vi "Configure Trigger.vi"(4 "impedence":enum16{"50 Ohm", "1 kOhm"}(ring), 6 "threshold (V)":dbl=1.0 min=0.9 max=1.6, 8 "error in (no error)":errorcluster, 9 "trigger source":T2, 10 "trigger mode":T1 items=["Single", "Continuous", "Gated", "Burst"], 11 "VISA resource name":refnum<visa-resource-name>) -> (0 "error out":errorcluster, 3 "VISA resource name out":refnum<visa-resource-name>)   [LabVIEW 2019, in "Pulse Rider PG-1000.lvlib"]
doc: "Configures the triggering settings of the instrument."
uses:
  <instrlib>/LV_PulseRiderPG1000/Pulse Rider PG-1000.lvlib
  <instrlib>/LV_PulseRiderPG1000/Public/Configure/Trigger/Trigger Source.ctl
  <instrlib>/LV_PulseRiderPG1000/Public/Configure/Trigger/Trigger Mode.ctl
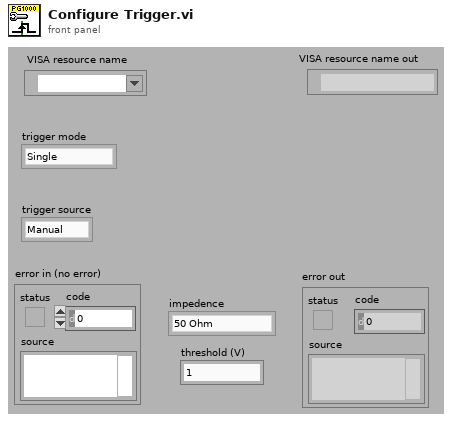
[diagram p1: front panel]
types:
  T1 = typedef "Pulse Rider PG-1000.lvlib/Trigger Mode.ctl" = u16
  T2 = typedef "Pulse Rider PG-1000.lvlib/Trigger Source.ctl" = enum16{"Manual", "External", "Timer"}
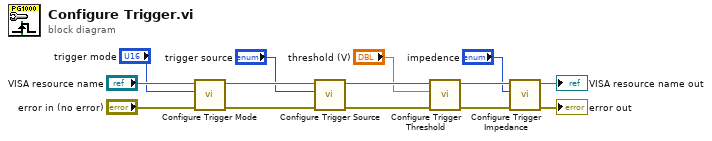
[diagram p0: block diagram]
diagram:
  n1 = call <instrlib>:"Configure Trigger Mode.vi"("error in (no error)"="error in (no error)", "trigger mode (Single)"="trigger mode", "VISA resource name"="VISA resource name") -> ("error out"=w13:errorcluster, "VISA resource name out"=w14:refnum<visa-resource-name>)  [unwired: 7 in]
  n2 = call <instrlib>:"Configure Trigger Source.vi"("error in (no error)"=w13, "trigger source"="trigger source", "VISA resource name"=w14) -> ("error out"=w11:errorcluster, "VISA resource name out"=w12:refnum<visa-resource-name>)  [unwired: 7 in]
  n3 = call <instrlib>:"Configure Trigger Threshold.vi"("error in (no error)"=w11, "threshold (V)"="threshold (V)", "VISA resource name"=w12) -> ("error out"=w9:errorcluster, "VISA resource name out"=w10:refnum<visa-resource-name>)  [unwired: 7 in]
  n4 = call <instrlib>:"Configure Trigger Impedance.vi"("error in (no error)"=w9, "impedence (50 Ohm)"="impedence", "VISA resource name"=w10) -> ("error out"=→"error out":errorcluster, "VISA resource name out"=→"VISA resource name out":refnum<visa-resource-name>)  [unwired: 7 in]
